vi "Disabled.vi"(7 "Robot Mode":T2, 10 "Match Info":T1={"Autonomous Elapsed Seconds"=0.0, "TeleOp Elapsed Seconds"=0.0, "Disabled Elapsed Seconds"=0.0, "Visited Autonomous"=FALSE, "Visited TeleOp"=FALSE, "Visited Disabled"=FALSE, "Autonomous Settings"={"Autonomous Style"=enum."Independent", "VI Refnum"=refnum}}, 11 "Call Context":T3) -> ()   [LabVIEW 2011]
doc: "This VI is called each time a disabled packet is received from the DS. It is often used to prepare for the next robot mode, to calibrate sensors, etc."
uses:
  <vilib>/Rock Robotics/WPI/DriverStation/WPI_DriverStationDerivedRobotMode.ctl
  <vilib>/Rock Robotics/WPI/DriverStation/WPI_DriverStationRobotMode.ctl
  <vilib>/Rock Robotics/WPI/DriverStation/WPI_DriverStationMatch Info.ctl
  <vilib>/Rock Robotics/WPI/CAN/Jaguar/SubVIs/WPI_CANJaguar_ControlMode.ctl
  <vilib>/Rock Robotics/WPI/CAN/Jaguar/SubVIs/WPI_CANJaguar_SpeedReference.ctl
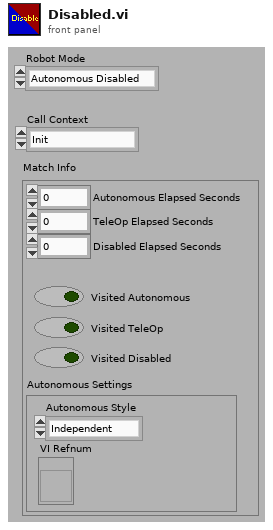
[diagram p1: front panel]
types:
  T1 = typedef "WPI_DriverStationMatch Info.ctl" = cluster{"Autonomous Elapsed Seconds":dbl, "TeleOp Elapsed Seconds":dbl, "Disabled Elapsed Seconds":dbl, "Visited Autonomous":bool, "Visited TeleOp":bool, "Visited Disabled":bool, "Autonomous Settings":cluster{"Autonomous Style":enum16{"Iterative", "Independent"}, "VI Refnum":refnum<vi>}}
  T2 = typedef "WPI_DriverStationRobotMode.ctl" = enum16{"Autonomous Disabled", "Autonomous Enabled", "Teleop Disabled", "Teleop Enabled", "Timeout", "Finish"}
  T3 = typedef "WPI_DriverStationDerivedRobotMode.ctl" = enum16{"Init", "Execute", "Stop"}
  T4 = typedef "WPI_CANJaguar_SpeedReference.ctl" = u8
  T5 = typedef "WPI_CANJaguar_ControlMode.ctl" = enum8{"Percent VBus", "Current", "Speed", "Position", "Voltage"}
  T6 = typedef "WPI_MotorControlDeviceRef.ctl" = cluster{"DeviceStatus":errorcluster, "Type":enum16{"PWM", "CAN"}, "PWM":cluster{"Digital Module":T7, "PWM Channel":T8, "DeadBand":T9}, "CAN":cluster{"Device Number":u8, "Control Mode":T5, "Semaphore":T10, "Max Vout":dbl}, "Invert":bool, "TransformRef":T11, "InvTransformRef":T11}
  T7 = typedef "FPGA_TypedefDigitalModule.ctl" = enum16{"Digital Module 1", "Digital Module 2"}
  T8 = typedef "FPGA_DIOPWMChannel.ctl" = enum8{"PWM 1", "PWM 2", "PWM 3", "PWM 4", "PWM 5", "PWM 6", "PWM 7", "PWM 8", "PWM 9", "PWM 10", "Invalid"}
  T9 = typedef "WPI_PWMDeadband.ctl" = cluster{"Name":string, "maxPositivePwm":i32, "minPositivePwm":i32, "centerPwm":i32, "maxNegativePwm":i32, "minNegativePwm":i32, "angularRange":u16}
  T10 = typedef "Semaphore RefNum" = refnum<k1>
  T11 = typedef "WPI_PWMTransform_ConPane.ctl" = refnum<vi>
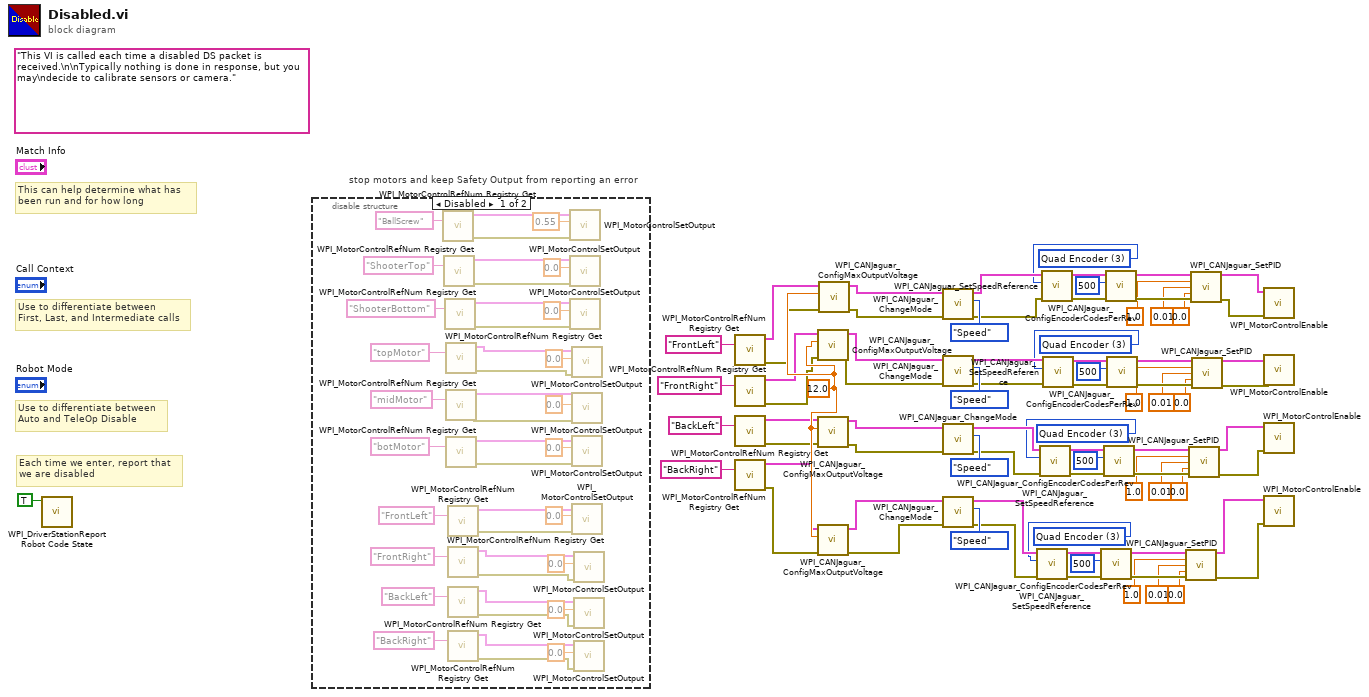
[diagram p0: block diagram]
diagram:
  w17 = T4 3 items=["Encoder"=0, "Inv Encoder"=2, "Quad Encoder"=3, "None"=255] ("Speed Reference")
  w18 = T4 3 items=["Encoder"=0, "Inv Encoder"=2, "Quad Encoder"=3, "None"=255] ("Speed Reference")
  w19 = T4 3 items=["Encoder"=0, "Inv Encoder"=2, "Quad Encoder"=3, "None"=255] ("Speed Reference")
  w20 = T4 3 items=["Encoder"=0, "Inv Encoder"=2, "Quad Encoder"=3, "None"=255] ("Speed Reference")
  w69 = 12.0 ("Maximum Output Voltage")
  (unwired) "This VI is called each time a disabled DS packet is received.\n\nTypically nothing is done in response, but you may\ndecide to calibrate sensors or camera."
  # "Each time we enter, report that\nwe are disabled"
  # "stop motors and keep Safety Output from reporting an error"
  # "Use to differentiate between\nFirst, Last, and Intermediate calls"
  # "This can help determine what has\nbeen run and for how long"
  # "Use to differentiate between\nAuto and TeleOp Disable"
  n1 = call <vilib>:"WPI_DriverStationReport Robot Code State.vi"("Disabled"=TRUE ("Autonomous")) -> ()  [unwired: 10 in, 1 out]
  n2 = disable-structure shown="Disabled" {
    frame Disabled {
      n3 = call <vilib>:"WPI_MotorControlRefNum Registry Get.vi"("refnum name"="BallScrew") -> ("error out"=w116:errorcluster, "MotorControlDevRef"=w117:T6)  [unwired: 9 in]
      n4 = call <vilib>:"WPI_MotorControlRefNum Registry Get.vi"("refnum name"="ShooterTop") -> ("error out"=w109:errorcluster, "MotorControlDevRef"=w112:T6)  [unwired: 9 in]
      n5 = call <vilib>:"WPI_MotorControlRefNum Registry Get.vi"("refnum name"="ShooterBottom") -> ("error out"=w110:errorcluster, "MotorControlDevRef"=w111:T6)  [unwired: 9 in]
      n6 = call <vilib>:"WPI_MotorControlRefNum Registry Get.vi"("refnum name"="topMotor") -> ("error out"=w102:errorcluster, "MotorControlDevRef"=w103:T6)  [unwired: 9 in]
      n7 = call <vilib>:"WPI_MotorControlRefNum Registry Get.vi"("refnum name"="midMotor") -> ("error out"=w100:errorcluster, "MotorControlDevRef"=w101:T6)  [unwired: 9 in]
      n8 = call <vilib>:"WPI_MotorControlRefNum Registry Get.vi"("refnum name"="botMotor") -> ("error out"=w98:errorcluster, "MotorControlDevRef"=w99:T6)  [unwired: 9 in]
      n9 = call <vilib>:"WPI_MotorControlRefNum Registry Get.vi"("refnum name"="FrontLeft") -> ("error out"=w89:errorcluster, "MotorControlDevRef"=w90:T6)  [unwired: 9 in]
      n10 = call <vilib>:"WPI_MotorControlRefNum Registry Get.vi"("refnum name"="FrontRight") -> ("error out"=w87:errorcluster, "MotorControlDevRef"=w88:T6)  [unwired: 9 in]
      n11 = call <vilib>:"WPI_MotorControlRefNum Registry Get.vi"("refnum name"="BackLeft") -> ("error out"=w85:errorcluster, "MotorControlDevRef"=w86:T6)  [unwired: 9 in]
      n12 = call <vilib>:"WPI_MotorControlRefNum Registry Get.vi"("refnum name"="BackRight") -> ("error out"=w83:errorcluster, "MotorControlDevRef"=w84:T6)  [unwired: 9 in]
      n13 = call <vilib>:"WPI_MotorControlSetOutput.vi"("error in (no error)"=w116, "Output"=0.55, "MotorControlDevRef"=w117) -> ()  [unwired: 7 in, 2 out]
      n14 = call <vilib>:"WPI_MotorControlSetOutput.vi"("error in (no error)"=w109, "Output"=0.0, "MotorControlDevRef"=w112) -> ()  [unwired: 7 in, 2 out]
      n15 = call <vilib>:"WPI_MotorControlSetOutput.vi"("error in (no error)"=w110, "Output"=0.0, "MotorControlDevRef"=w111) -> ()  [unwired: 7 in, 2 out]
      n16 = call <vilib>:"WPI_MotorControlSetOutput.vi"("error in (no error)"=w102, "Output"=0.0, "MotorControlDevRef"=w103) -> ()  [unwired: 7 in, 2 out]
      n17 = call <vilib>:"WPI_MotorControlSetOutput.vi"("error in (no error)"=w100, "Output"=0.0, "MotorControlDevRef"=w101) -> ()  [unwired: 7 in, 2 out]
      n18 = call <vilib>:"WPI_MotorControlSetOutput.vi"("error in (no error)"=w98, "Output"=0.0, "MotorControlDevRef"=w99) -> ()  [unwired: 7 in, 2 out]
      n19 = call <vilib>:"WPI_MotorControlSetOutput.vi"("error in (no error)"=w89, "Output"=0.0, "MotorControlDevRef"=w90) -> ()  [unwired: 7 in, 2 out]
      n20 = call <vilib>:"WPI_MotorControlSetOutput.vi"("error in (no error)"=w87, "Output"=0.0, "MotorControlDevRef"=w88) -> ()  [unwired: 7 in, 2 out]
      n21 = call <vilib>:"WPI_MotorControlSetOutput.vi"("error in (no error)"=w85, "Output"=0.0, "MotorControlDevRef"=w86) -> ()  [unwired: 7 in, 2 out]
      n22 = call <vilib>:"WPI_MotorControlSetOutput.vi"("error in (no error)"=w83, "Output"=0.0, "MotorControlDevRef"=w84) -> ()  [unwired: 7 in, 2 out]
    }
    frame Enabled {
    }
  }
  n23 = call <vilib>:"WPI_MotorControlRefNum Registry Get.vi"("refnum name"="FrontLeft") -> ("error out"=w5:errorcluster, "MotorControlDevRef"=w12:T6)  [unwired: 9 in]
  n24 = call <vilib>:"WPI_MotorControlRefNum Registry Get.vi"("refnum name"="FrontRight") -> ("error out"=w6:errorcluster, "MotorControlDevRef"=w11:T6)  [unwired: 9 in]
  n25 = call <vilib>:"WPI_MotorControlRefNum Registry Get.vi"("refnum name"="BackLeft") -> ("error out"=w7:errorcluster, "MotorControlDevRef"=w10:T6)  [unwired: 9 in]
  n26 = call <vilib>:"WPI_MotorControlRefNum Registry Get.vi"("refnum name"="BackRight") -> ("error out"=w8:errorcluster, "MotorControlDevRef"=w9:T6)  [unwired: 9 in]
  n27 = call <vilib>:"WPI_CANJaguar_ConfigMaxOutputVoltage.vi"("error in (no error)"=w6, "Maximum Output Voltage"=w69, "CAN Jaguar Ref"=w11) -> ("error out"=w3:errorcluster, "CAN Jaguar Ref Out"=w71:T6)  [unwired: 7 in]
  n28 = call <vilib>:"WPI_CANJaguar_ConfigMaxOutputVoltage.vi"("error in (no error)"=w7, "Maximum Output Voltage"=w69, "CAN Jaguar Ref"=w10) -> ("error out"=w2:errorcluster, "CAN Jaguar Ref Out"=w72:T6)  [unwired: 7 in]
  n29 = call <vilib>:"WPI_CANJaguar_ConfigMaxOutputVoltage.vi"("error in (no error)"=w8, "Maximum Output Voltage"=w69, "CAN Jaguar Ref"=w9) -> ("error out"=w1:errorcluster, "CAN Jaguar Ref Out"=w73:T6)  [unwired: 7 in]
  n30 = call <vilib>:"WPI_CANJaguar_ConfigMaxOutputVoltage.vi"("error in (no error)"=w5, "Maximum Output Voltage"=w69, "CAN Jaguar Ref"=w12) -> ("error out"=w4:errorcluster, "CAN Jaguar Ref Out"=w70:T6)  [unwired: 7 in]
  n31 = call <vilib>:"WPI_CANJaguar_ChangeMode.vi"("error in (no error)"=w4, "Control Mode"=WPI_CANJaguar_ControlMode."Speed", "CAN Jaguar Ref"=w70) -> ("error out"=w34:errorcluster, "CAN Jaguar Ref Out"=w36:T6)  [unwired: 7 out]
  n32 = call <vilib>:"WPI_CANJaguar_ChangeMode.vi"("error in (no error)"=w3, "Control Mode"=WPI_CANJaguar_ControlMode."Speed", "CAN Jaguar Ref"=w71) -> ("error out"=w33:errorcluster, "CAN Jaguar Ref Out"=w35:T6)  [unwired: 7 out]
  n33 = call <vilib>:"WPI_CANJaguar_ChangeMode.vi"("error in (no error)"=w2, "Control Mode"=WPI_CANJaguar_ControlMode."Speed", "CAN Jaguar Ref"=w72) -> ("error out"=w31:errorcluster, "CAN Jaguar Ref Out"=w32:T6)  [unwired: 7 out]
  n34 = call <vilib>:"WPI_CANJaguar_ChangeMode.vi"("error in (no error)"=w1, "Control Mode"=WPI_CANJaguar_ControlMode."Speed", "CAN Jaguar Ref"=w73) -> ("error out"=w29:errorcluster, "CAN Jaguar Ref Out"=w30:T6)  [unwired: 7 out]
  n35 = call <vilib>:"WPI_CANJaguar_SetSpeedReference.vi"("error in (no error)"=w29, "Speed Reference"=w17, "CAN Jaguar Ref"=w30) -> ("error out"=w39:errorcluster, "CAN Jaguar Ref Out"=w38:T6)  [unwired: 7 in]
  n36 = call <vilib>:"WPI_CANJaguar_SetSpeedReference.vi"("error in (no error)"=w31, "Speed Reference"=w18, "CAN Jaguar Ref"=w32) -> ("error out"=w47:errorcluster, "CAN Jaguar Ref Out"=w46:T6)  [unwired: 7 in]
  n37 = call <vilib>:"WPI_CANJaguar_SetSpeedReference.vi"("error in (no error)"=w34, "Speed Reference"=w20, "CAN Jaguar Ref"=w36) -> ("error out"=w63:errorcluster, "CAN Jaguar Ref Out"=w62:T6)  [unwired: 7 in]
  n38 = call <vilib>:"WPI_CANJaguar_SetSpeedReference.vi"("error in (no error)"=w33, "Speed Reference"=w19, "CAN Jaguar Ref"=w35) -> ("error out"=w55:errorcluster, "CAN Jaguar Ref Out"=w54:T6)  [unwired: 7 in]
  n39 = call <vilib>:"WPI_CANJaguar_ConfigEncoderCodesPerRev.vi"("error in (no error)"=w39, "Encoder Codes Per Rev"=u16 500, "CAN Jaguar Ref"=w38) -> ("error out"=w43:errorcluster, "CAN Jaguar Ref Out"=w37:T6)  [unwired: 7 in]
  n40 = call <vilib>:"WPI_CANJaguar_ConfigEncoderCodesPerRev.vi"("error in (no error)"=w47, "Encoder Codes Per Rev"=u16 500, "CAN Jaguar Ref"=w46) -> ("error out"=w51:errorcluster, "CAN Jaguar Ref Out"=w45:T6)  [unwired: 7 in]
  n41 = call <vilib>:"WPI_CANJaguar_ConfigEncoderCodesPerRev.vi"("error in (no error)"=w63, "Encoder Codes Per Rev"=u16 500, "CAN Jaguar Ref"=w62) -> ("error out"=w67:errorcluster, "CAN Jaguar Ref Out"=w61:T6)  [unwired: 7 in]
  n42 = call <vilib>:"WPI_CANJaguar_ConfigEncoderCodesPerRev.vi"("error in (no error)"=w55, "Encoder Codes Per Rev"=u16 500, "CAN Jaguar Ref"=w54) -> ("error out"=w59:errorcluster, "CAN Jaguar Ref Out"=w53:T6)  [unwired: 7 in]
  n43 = call <vilib>:"WPI_CANJaguar_SetPID.vi"("CAN Jaguar Ref"=w37, "P"=1.0, "I"=0.01, "D"=0.0, "error in (no error)"=w43) -> ("CAN Jaguar Ref Out"=w22:T6, "error out"=w21:errorcluster)  [unwired: 9 in]
  n44 = call <vilib>:"WPI_CANJaguar_SetPID.vi"("CAN Jaguar Ref"=w45, "P"=1.0, "I"=0.01, "D"=0.0, "error in (no error)"=w51) -> ("CAN Jaguar Ref Out"=w24:T6, "error out"=w23:errorcluster)  [unwired: 9 in]
  n45 = call <vilib>:"WPI_CANJaguar_SetPID.vi"("CAN Jaguar Ref"=w61, "P"=1.0, "I"=0.01, "D"=0.0, "error in (no error)"=w67) -> ("CAN Jaguar Ref Out"=w25:T6, "error out"=w26:errorcluster)  [unwired: 9 in]
  n46 = call <vilib>:"WPI_CANJaguar_SetPID.vi"("CAN Jaguar Ref"=w53, "P"=1.0, "I"=0.01, "D"=0.0, "error in (no error)"=w59) -> ("CAN Jaguar Ref Out"=w28:T6, "error out"=w27:errorcluster)  [unwired: 9 in]
  n47 = call <vilib>:"WPI_MotorControlEnable.vi"("error in (no error)"=w26, "CAN Jaguar Ref"=w25) -> ()  [unwired: 1 in, 9 out]
  n48 = call <vilib>:"WPI_MotorControlEnable.vi"("error in (no error)"=w27, "CAN Jaguar Ref"=w28) -> ()  [unwired: 1 in, 9 out]
  n49 = call <vilib>:"WPI_MotorControlEnable.vi"("error in (no error)"=w23, "CAN Jaguar Ref"=w24) -> ()  [unwired: 1 in, 9 out]
  n50 = call <vilib>:"WPI_MotorControlEnable.vi"("error in (no error)"=w21, "CAN Jaguar Ref"=w22) -> ()  [unwired: 1 in, 9 out]
